vi "Parse Member.vi"(8 "error in (no error)":errorcluster, 10 "member":string, 11 "ARN in":refnum<class "ARN.lvclass">) -> (0 "error out":errorcluster, 3 "ARN out":refnum<class "ARN.lvclass">)   [LabVIEW 2015, in "NI_AWS_Core.lvlib" / "ARN.lvclass"]
uses:
  ARN.lvclass
  ARN.lvclass/ARN.ctl
  Write ARN.vi
  HTTP Request/HTTP Request.lvclass
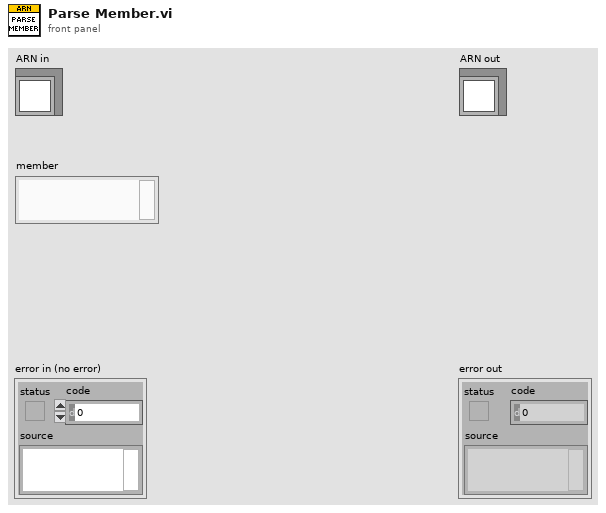
[diagram p1: front panel]
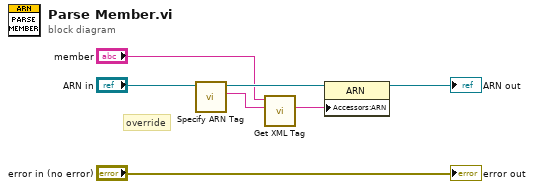
[diagram p0: block diagram]
diagram:
  # "override"
  n1 = call-dynamic "Specify ARN Tag.vi"("ARN in"="ARN in") -> ("ARN Tag"=w4:string, "ARN out"=w5:refnum<class "ARN.lvclass">)  [unwired: 9 in]
  n2 = call "Get XML Tag.vi"("Tag name"=w4, "XML String in"="member") -> ("Tag value"=w6:string)  [unwired: 5 in, 4 out]
  n3 = property class="ARN"(reference=w5, "Accessors:ARN"=w6) -> (reference out=→"ARN out":refnum<class "ARN.lvclass">)  [unwired: 1 in, 1 out]
  "error out" <- "error in (no error)"
